vi "LSMcontroller_v61_updatedROIselection.vi"() -> ()   [LabVIEW 2015] (continued)
                    n4179 = local read "srateAODOtt"() -> (w920:dbl)
                    n4180 = local read "srateAODOtt"() -> (w927:dbl)
                    n4181 = local read "continuous"() -> (w932:bool)
                    n4182 = local read "Angle ref"() -> (w917:dbl)
                    n4183 = local read "wavdet"() -> (w934:bool)
                    n4184 = local read "Vx-ref"() -> (w929:dbl)
                    n4185 = local read "Vy-ref"() -> (w931:dbl)
                    n4186 = local read "avpp"() -> (w930:i32)
                    n4187 = call "tt_timeandsamples.vi"("bin"=w924, "refreshtime"=w918, "srateAODOtt"=w921, "tot#ofsamples"=w926) -> ("refreshrate"=w922:dbl, "refreshbuffer"=w923:i32, "timetracecycles"=w928:i32)  [unwired: 5 in]
                    n4188 = local read "bin"() -> (w925:dbl)
                    n4189 = call "2pparameters.vi"("command"="get") -> ("params out"=w937:T11)  [unwired: 1 in]
                    n4190 = Bundle By Name(cluster=w937, "Drawing Mode"=w910, "measpoints"=w926, "tt_cycles"=w928, "refreshbuffer"=w923, "refreshrate"=w922, "Vx-ref"=w929, "Vy-ref"=w931, "srate"=w920, "finite"=w933, "cont"=w932, "wavdet"=w934, "avpp"=w930, "srateAODO"=w927, "bufferAI"=w923, "bin"=w925, "Angle Img"=w917, "Vxminref"=w916, "Vxmaxref"=w915, "Vyminref"=w914, "Vymaxref"=w913, "Xpixels Img"=w912, "Ypixels Img"=w911, "Pel"=w909, "Vz-reset"=0.0, "AIoverride"=w907, "type"="Lifetime (contour)") -> (w935:T11)
                    n4191 = Reciprocal(x=w922) -> (1/x=w919:dbl)
                    n4192 = local write "refreshtime"(w919) -> ()
                    n4193 = call "2pparameters.vi"("Params in"=w935, "command"="set") -> ()  [unwired: 1 out]
                  }
                  frame "X-Y-Z-t movie" {
                  }
                  frame "linescan" {
                  }
                  frame "Timetrace" {
                    n4194 = local read "Vy-min draw"() -> (w947:dbl)
                    n4195 = local read "Vy-max draw"() -> (w946:dbl)
                    n4196 = local read "Vx-min draw"() -> (w949:dbl)
                    n4197 = local read "Vx-max draw"() -> (w948:dbl)
                    n4198 = local read "xpixels ref"() -> (w945:i32)
                    n4199 = local read "ypixels ref"() -> (w944:i32)
                    n4200 = local read "ROI Type"() -> (w943:u16)
                    n4201 = local read "srateAODOtt"() -> (w954:dbl)
                    n4202 = local read "# of frames"() -> (w959:i32)
                    n4203 = local read "refreshtime"() -> (w951:dbl)
                    n4204 = local read "Pel"() -> (w942:dbl)
                    n4205 = local read "bin"() -> (w957:dbl)
                    n4206 = local read "Override AI buffer"() -> (w940:bool)
                    n4207 = local read "finite samples"() -> (w966:bool)
                    n4208 = local read "srateAODOtt"() -> (w953:dbl)
                    n4209 = local read "srateAODOtt"() -> (w960:dbl)
                    n4210 = local read "continuous"() -> (w965:bool)
                    n4211 = local read "Angle ref"() -> (w950:dbl)
                    n4212 = local read "wavdet"() -> (w967:bool)
                    n4213 = local read "Vx-ref"() -> (w962:dbl)
                    n4214 = local read "Vy-ref"() -> (w964:dbl)
                    n4215 = local read "avpp"() -> (w963:i32)
                    n4216 = call "tt_timeandsamples.vi"("bin"=w957, "refreshtime"=w951, "srateAODOtt"=w954, "tot#ofsamples"=w959) -> ("refreshrate"=w955:dbl, "refreshbuffer"=w956:i32, "timetracecycles"=w961:i32)  [unwired: 5 in]
                    n4217 = local read "bin"() -> (w958:dbl)
                    n4218 = call "2pparameters.vi"("command"="get") -> ("params out"=w970:T11)  [unwired: 1 in]
                    n4219 = Bundle By Name(cluster=w970, "Drawing Mode"=w943, "measpoints"=w959, "tt_cycles"=w961, "refreshbuffer"=w956, "refreshrate"=w955, "Vx-ref"=w962, "Vy-ref"=w964, "srate"=w953, "finite"=w966, "cont"=w965, "wavdet"=w967, "avpp"=w963, "srateAODO"=w960, "bufferAI"=w956, "bin"=w958, "Angle Img"=w950, "Vxminref"=w949, "Vxmaxref"=w948, "Vyminref"=w947, "Vymaxref"=w946, "Xpixels Img"=w945, "Ypixels Img"=w944, "Pel"=w942, "Vz-reset"=0.0, "AIoverride"=w940, "type"="Timetrace") -> (w968:T11)
                    n4220 = Reciprocal(x=w955) -> (1/x=w952:dbl)
                    n4221 = local write "refreshtime"(w952) -> ()
                    n4222 = call "2pparameters.vi"("Params in"=w968, "command"="set") -> ()  [unwired: 1 out]
                  }
                  frame "Lifetime (point)" {
                  }
                }
              }
              frame #1 {
                w973 = FALSE ("wavdet")
                n4223 = call "2pparameters.vi"("command"="get") -> ("params out"=w977:T11)  [unwired: 1 in]
                n4224 = Bundle By Name(cluster=w977, "finite"=w973, "cont"=w973, "wavdet"=TRUE) -> (w974:T11)
                n4225 = call "2pparameters.vi"("Params in"=w974, "command"="set") -> ()  [unwired: 1 out]
              }
              frame #2 {
                n4226 = local read "DO channels"() -> (w982:u16)
                n4227 = call "2pparameters.vi"("command"="get") -> ("params out"=w984:T11)  [unwired: 1 in]
                n4228 = Unbundle By Name(w984) -> ("aDO"=w983:u32[])
                n4229 = Search 1D Array(1D array=w983, element=w982) -> (index of element=w980:i32)  [unwired: 1 in]
                n4230 = Greater?(x=w980, y=-1) -> (0:w979:bool)
                n4231 = case shown="True" w979 {
                  tunnel: w980 -> [_ w993]
                  frame False {
                  }
                  frame True {
                    n4232 = local read "Meastab"() -> (w987:enum32{"X-Y Image", "Linescan", "Timetrace"})
                    n4233 = local read "Digital padding value"() -> (w988:dbl)
                    n4234 = local read "Digital time offset (s)"() -> (w989:dbl)
                    n4235 = case shown="\"Timetrace\"" w987 {
                      tunnel: [w994 w995] -> w986
                      frame "X-Y Image", Default {
                        n4236 = local read "Sampling rate"() -> (w994:dbl)
                      }
                      frame "Timetrace" {
                        n4237 = local read "srateAODOtt"() -> (w995:dbl)
                      }
                    }
                    n4238 = local read "Digital Freq (Hz)"() -> (w991:dbl)
                    n4239 = local read "Digital phase (s)"() -> (w990:dbl)
                    n4240 = local read "Digital DC (%)"() -> (w992:dbl)
                    n4241 = call "replace DO wf param.vi"("Digital Freq (Hz)"=w991, "Digital DC (%)"=w992, "Digital phase"=w990, "Sampling frequency (Hz)"=w986, "Digital time offset (s)"=w989, "index of DO wave"=w993, "padding value"=w988) -> ()  [unwired: 4 in]
                  }
                }
              }
              frame #3 {
                n4242 = case shown="True" w996 {
                  tunnel: w997 -> [_ w1004]
                  frame False {
                  }
                  frame True {
                    n4243 = local read "Meastab"() -> (w1001:enum32{"X-Y Image", "Linescan", "Timetrace"})
                    n4244 = call "waveformparamsv2.vi"("command"="get") -> ("Params out"=w1020:T15)  [unwired: 4 in, 2 out]
                    n4245 = Unbundle By Name(w1020) -> ("DO parameters"=w1019:T18)
                    n4246 = property on="refwf" class="Ring (strict)"() -> ("RingText.Text"=w1026:string)  [unwired: 2 in, 2 out]
                    n4247 = case shown="\"Timetrace\"" w1001 {
                      tunnel: [w1027 w1028] -> w1000
                      frame "X-Y Image", Default {
                        n4248 = local read "Sampling rate"() -> (w1027:dbl)
                      }
                      frame "Timetrace" {
                        n4249 = local read "srateAODOtt"() -> (w1028:dbl)
                      }
                    }
                    n4250 = call "waveformsAObuffer.vi"("command"="get") -> ("AO wf out"=w1024:waveform(dbl)[])  [unwired: 1 in]
                    n4251 = call "waveformsDObuffer.vi"("command"="get") -> ("DO wf out"=w1022:digitalwaveform[])  [unwired: 1 in]
                    n4252 = call "referfencesize.vi"("Digital waveforms in"=w1022, "Analog waveforms in"=w1024, "reference waveforms to"=w1026) -> ("number of samples"=w1017:i32)  [unwired: 2 in]
                    n4253 = Index Array(array=w1019, index=w1004) -> (element=w1018:T19)
                    n4254 = call "waveformsDObuffer.vi"("command"="get") -> ("DO wf out"=w1014:digitalwaveform[])  [unwired: 1 in]
                    n4255 = call "simple digital from wf params.vi"("waveform params"=w1018, "number of samples"=w1017) -> ("digital waveform"=w1016:digitalwaveform)
                    n4256 = property on="refwf" class="Ring (strict)"() -> ("RingText.Text"=w1006:string)  [unwired: 2 in, 2 out]
                    n4257 = Replace Array Subset(array=w1014, new element=w1016, index=w1004) -> (w1005:digitalwaveform[])
                    n4258 = call "waveformsAObuffer.vi"("command"="get") -> ("AO wf out"=w1013:waveform(dbl)[])  [unwired: 1 in]
                    n4259 = local read "wavdet"() -> (w1003:bool)
                    n4260 = call "correctwaveformsizetemp.vi"("new sampling frequency (Hz)"=w1000, "start"=FALSE, "reference waveforms to"=w1006, "Analog waveforms in"=w1013, "stop"=FALSE, "Digital waveforms in"=w1005) -> ("analog wf out"=w1009:waveform(dbl)[], "Digital wf out"=w1007:digitalwaveform[], "measpoints"=w1002:i32)
                    n4261 = local write "Analog Lines Plot"(w1009) -> ()
                    n4262 = call "GetNumCamFramesv2.vi"("Digital Waveform Graph"=w1007) -> ("Numeric"=w1008:i32)  [unwired: 10 in]
                    n4263 = local write "Digital Lines Plot"(w1007) -> ()
                    n4264 = case shown="True" w1003 {
                      tunnel: w1002 -> [_ w1029]
                      frame False {
                      }
                      frame True {
                        n4265 = local write "# of frames"(w1029) -> ()
                      }
                    }
                    n4266 = call "waveformsAObuffer.vi"("AO wf in"=w1009, "command"="set") -> ()  [unwired: 1 out]
                    n4267 = call "waveformsDObuffer.vi"("DO wf in"=w1007, "command"="set") -> ()  [unwired: 1 out]
                    n4268 = local write "Total Camera Frames"(w1008) -> ()
                  }
                }
              }
              frame #4 {
                n4269 = local read "finite samples"() -> (w1030:bool)
                n4270 = local read "continuous"() -> (w1031:bool)
                n4271 = local read "wavdet"() -> (w1032:bool)
                n4272 = call "2pparameters.vi"("command"="get") -> ("params out"=w1035:T11)  [unwired: 1 in]
                n4273 = Bundle By Name(cluster=w1035, "finite"=w1030, "cont"=w1031, "wavdet"=w1032) -> (w1033:T11)
                n4274 = call "2pparameters.vi"("Params in"=w1033, "command"="set") -> ()  [unwired: 1 out]
              }
            }
          }
          event "refwf": Value Change {
            n4275 = event-data() -> ()  [unwired: 1 in, 6 out]
            n4276 = stacked-sequence {
              frame #0 {
                n4277 = local read "Measurement"() -> (w1037:T4)
                n4278 = case shown="\"X-Y-t movie\", Default" w1037 {
                  frame "X-Y-t movie", Default {
                    n4279 = local read "avpp"() -> (w1058:i32)
                    n4280 = local read "Angle ref"() -> (w1057:dbl)
                    n4281 = local read "ROI Type"() -> (w1056:u16)
                    n4282 = local read "xpixels ref"() -> (w1053:i32)
                    n4283 = local read "Vx-min ref"() -> (w1052:dbl)
                    n4284 = local read "Vx-max ref"() -> (w1051:dbl)
                    n4285 = local read "ypixels ref"() -> (w1049:i32)
                    n4286 = local read "Vy-min ref"() -> (w1050:dbl)
                    n4287 = local read "Vy-max ref"() -> (w1046:dbl)
                    n4288 = local read "Sampling rate"() -> (w1040:dbl)
                    n4289 = local read "finite samples"() -> (w1041:bool)
                    n4290 = local read "continuous"() -> (w1044:bool)
                    n4291 = local read "wavdet"() -> (w1045:bool)
                    n4292 = local read "# of frames"() -> (w1043:i32)
                    n4293 = local read "maxbufferAI"() -> (w1042:i32)
                    n4294 = local read "Override AI buffer"() -> (w1038:bool)
                    n4295 = call "2pparameters.vi"("command"="get") -> ("params out"=w1055:T11)  [unwired: 1 in]
                    n4296 = Bundle By Name(cluster=w1055, "type"="X-Y-t movie", "avpp"=w1058, "Angle Img"=w1057, "Xpixels Img"=w1053, "Vx-min Img"=w1052, "VX-max Img"=w1051, "Ypixels Img"=w1049, "Vy-min Img"=w1050, "Vy-max Img"=w1046, "srate"=w1040, "srate Img"=w1040, "finite"=w1041, "cont"=w1044, "wavdet"=w1045, "measpoints"=w1043, "maxbufferAI"=w1042, "Drawing Mode"=w1056, "Vz-reset"=0.0, "AIoverride"=w1038) -> (w1047:T11)
                    n4297 = call "2pparameters.vi"("Params in"=w1047, "command"="set") -> ()  [unwired: 1 out]
                  }
                  frame "X-Y-Z stack" {
                    n4298 = call "2pparameters.vi"("command"="get") -> ("params out"=w1062:T11)  [unwired: 1 in]
                    n4299 = Bundle By Name(cluster=w1062, "type"="X-Y-Z stack") -> (w1060:T11)
                    n4300 = call "2pparameters.vi"("Params in"=w1060, "command"="set") -> ()  [unwired: 1 out]
                  }
                  frame "Lifetime (scan)" {
                    n4301 = call "2pparameters.vi"("command"="get") -> ("params out"=w1067:T11)  [unwired: 1 in]
                    n4302 = Bundle By Name(cluster=w1067, "type"="Lifetime (scan)") -> (w1065:T11)
                    n4303 = call "2pparameters.vi"("Params in"=w1065, "command"="set") -> ()  [unwired: 1 out]
                  }
                  frame "Lifetime (contour)" {
                    n4304 = local read "Vy-min draw"() -> (w1077:dbl)
                    n4305 = local read "Vy-max draw"() -> (w1076:dbl)
                    n4306 = local read "Vx-min draw"() -> (w1079:dbl)
                    n4307 = local read "Vx-max draw"() -> (w1078:dbl)
                    n4308 = local read "xpixels ref"() -> (w1075:i32)
                    n4309 = local read "ypixels ref"() -> (w1074:i32)
                    n4310 = local read "ROI Type"() -> (w1073:u16)
                    n4311 = local read "srateAODOtt"() -> (w1084:dbl)
                    n4312 = local read "# of frames"() -> (w1089:i32)
                    n4313 = local read "refreshtime"() -> (w1081:dbl)
                    n4314 = local read "Pel"() -> (w1072:dbl)
                    n4315 = local read "bin"() -> (w1087:dbl)
                    n4316 = local read "Override AI buffer"() -> (w1070:bool)
                    n4317 = local read "finite samples"() -> (w1096:bool)
                    n4318 = local read "srateAODOtt"() -> (w1083:dbl)
                    n4319 = local read "srateAODOtt"() -> (w1090:dbl)
                    n4320 = local read "continuous"() -> (w1095:bool)
                    n4321 = local read "Angle ref"() -> (w1080:dbl)
                    n4322 = local read "wavdet"() -> (w1097:bool)
                    n4323 = local read "Vx-ref"() -> (w1092:dbl)
                    n4324 = local read "Vy-ref"() -> (w1094:dbl)
                    n4325 = local read "avpp"() -> (w1093:i32)
                    n4326 = call "tt_timeandsamples.vi"("bin"=w1087, "refreshtime"=w1081, "srateAODOtt"=w1084, "tot#ofsamples"=w1089) -> ("refreshrate"=w1085:dbl, "refreshbuffer"=w1086:i32, "timetracecycles"=w1091:i32)  [unwired: 5 in]
                    n4327 = local read "bin"() -> (w1088:dbl)
                    n4328 = call "2pparameters.vi"("command"="get") -> ("params out"=w1100:T11)  [unwired: 1 in]
                    n4329 = Bundle By Name(cluster=w1100, "Drawing Mode"=w1073, "measpoints"=w1089, "tt_cycles"=w1091, "refreshbuffer"=w1086, "refreshrate"=w1085, "Vx-ref"=w1092, "Vy-ref"=w1094, "srate"=w1083, "finite"=w1096, "cont"=w1095, "wavdet"=w1097, "avpp"=w1093, "srateAODO"=w1090, "bufferAI"=w1086, "bin"=w1088, "Angle Img"=w1080, "Vxminref"=w1079, "Vxmaxref"=w1078, "Vyminref"=w1077, "Vymaxref"=w1076, "Xpixels Img"=w1075, "Ypixels Img"=w1074, "Pel"=w1072, "Vz-reset"=0.0, "AIoverride"=w1070, "type"="Lifetime (contour)") -> (w1098:T11)
                    n4330 = Reciprocal(x=w1085) -> (1/x=w1082:dbl)
                    n4331 = local write "refreshtime"(w1082) -> ()
                    n4332 = call "2pparameters.vi"("Params in"=w1098, "command"="set") -> ()  [unwired: 1 out]
                  }
                  frame "X-Y-Z-t movie" {
                  }
                  frame "linescan" {
                  }
                  frame "Timetrace" {
                    n4333 = local read "Vy-min draw"() -> (w1110:dbl)
                    n4334 = local read "Vy-max draw"() -> (w1109:dbl)
                    n4335 = local read "Vx-min draw"() -> (w1112:dbl)
                    n4336 = local read "Vx-max draw"() -> (w1111:dbl)
                    n4337 = local read "xpixels ref"() -> (w1108:i32)
                    n4338 = local read "ypixels ref"() -> (w1107:i32)
                    n4339 = local read "ROI Type"() -> (w1106:u16)
                    n4340 = local read "srateAODOtt"() -> (w1117:dbl)
                    n4341 = local read "# of frames"() -> (w1122:i32)
                    n4342 = local read "refreshtime"() -> (w1114:dbl)
                    n4343 = local read "Pel"() -> (w1105:dbl)
                    n4344 = local read "bin"() -> (w1120:dbl)
                    n4345 = local read "Override AI buffer"() -> (w1103:bool)
                    n4346 = local read "finite samples"() -> (w1129:bool)
                    n4347 = local read "srateAODOtt"() -> (w1116:dbl)
                    n4348 = local read "srateAODOtt"() -> (w1123:dbl)
                    n4349 = local read "continuous"() -> (w1128:bool)
                    n4350 = local read "Angle ref"() -> (w1113:dbl)
                    n4351 = local read "wavdet"() -> (w1130:bool)
                    n4352 = local read "Vx-ref"() -> (w1125:dbl)
                    n4353 = local read "Vy-ref"() -> (w1127:dbl)
                    n4354 = local read "avpp"() -> (w1126:i32)
                    n4355 = call "tt_timeandsamples.vi"("bin"=w1120, "refreshtime"=w1114, "srateAODOtt"=w1117, "tot#ofsamples"=w1122) -> ("refreshrate"=w1118:dbl, "refreshbuffer"=w1119:i32, "timetracecycles"=w1124:i32)  [unwired: 5 in]
                    n4356 = local read "bin"() -> (w1121:dbl)
                    n4357 = call "2pparameters.vi"("command"="get") -> ("params out"=w1133:T11)  [unwired: 1 in]
                    n4358 = Bundle By Name(cluster=w1133, "Drawing Mode"=w1106, "measpoints"=w1122, "tt_cycles"=w1124, "refreshbuffer"=w1119, "refreshrate"=w1118, "Vx-ref"=w1125, "Vy-ref"=w1127, "srate"=w1116, "finite"=w1129, "cont"=w1128, "wavdet"=w1130, "avpp"=w1126, "srateAODO"=w1123, "bufferAI"=w1119, "bin"=w1121, "Angle Img"=w1113, "Vxminref"=w1112, "Vxmaxref"=w1111, "Vyminref"=w1110, "Vymaxref"=w1109, "Xpixels Img"=w1108, "Ypixels Img"=w1107, "Pel"=w1105, "Vz-reset"=0.0, "AIoverride"=w1103, "type"="Timetrace") -> (w1131:T11)
                    n4359 = Reciprocal(x=w1118) -> (1/x=w1115:dbl)
                    n4360 = local write "refreshtime"(w1115) -> ()
                    n4361 = call "2pparameters.vi"("Params in"=w1131, "command"="set") -> ()  [unwired: 1 out]
                  }
                  frame "Lifetime (point)" {
                  }
                }
              }
              frame #1 {
                w1136 = FALSE ("wavdet")
                n4362 = call "2pparameters.vi"("command"="get") -> ("params out"=w1140:T11)  [unwired: 1 in]
                n4363 = Bundle By Name(cluster=w1140, "finite"=w1136, "cont"=w1136, "wavdet"=TRUE) -> (w1137:T11)
                n4364 = call "2pparameters.vi"("Params in"=w1137, "command"="set") -> ()  [unwired: 1 out]
              }
              frame #2 {
                n4365 = local read "Meastab"() -> (w1145:enum32{"X-Y Image", "Linescan", "Timetrace"})
                n4366 = property on="refwf" class="Ring (strict)"() -> ("RingText.Text"=w1148:string)  [unwired: 2 in, 2 out]
                n4367 = case shown="\"Timetrace\"" w1145 {
                  tunnel: [w1158 w1159] -> w1144
                  frame "X-Y Image", Default {
                    n4368 = local read "Sampling rate"() -> (w1158:dbl)
                  }
                  frame "Timetrace" {
                    n4369 = local read "srateAODOtt"() -> (w1159:dbl)
                  }
                }
                n4370 = call "waveformsAObuffer.vi"("command"="get") -> ("AO wf out"=w1157:waveform(dbl)[])  [unwired: 1 in]
                n4371 = local read "wavdet"() -> (w1147:bool)
                n4372 = call "waveformsDObuffer.vi"("command"="get") -> ("DO wf out"=w1153:digitalwaveform[])  [unwired: 1 in]
                n4373 = call "correctwaveformsizetemp.vi"("new sampling frequency (Hz)"=w1144, "start"=FALSE, "reference waveforms to"=w1148, "Analog waveforms in"=w1157, "stop"=FALSE, "Digital waveforms in"=w1153) -> ("analog wf out"=w1151:waveform(dbl)[], "Digital wf out"=w1149:digitalwaveform[], "measpoints"=w1146:i32)
                n4374 = local write "Analog Lines Plot"(w1151) -> ()
                n4375 = call "GetNumCamFramesv2.vi"("Digital Waveform Graph"=w1149) -> ("Numeric"=w1150:i32)  [unwired: 10 in]
                n4376 = local write "Digital Lines Plot"(w1149) -> ()
                n4377 = call "waveformsDObuffer.vi"("DO wf in"=w1149, "command"="set") -> ()  [unwired: 1 out]
                n4378 = call "waveformsAObuffer.vi"("AO wf in"=w1151, "command"="set") -> ()  [unwired: 1 out]
                n4379 = local write "Total Camera Frames"(w1150) -> ()
                n4380 = case shown="True" w1147 {
                  tunnel: w1146 -> [_ w1160]
                  frame False {
                  }
                  frame True {
                    n4381 = local write "# of frames"(w1160) -> ()
                  }
                }
              }
              frame #3 {
                n4382 = local read "finite samples"() -> (w1161:bool)
                n4383 = local read "continuous"() -> (w1162:bool)
                n4384 = local read "wavdet"() -> (w1163:bool)
                n4385 = call "2pparameters.vi"("command"="get") -> ("params out"=w1166:T11)  [unwired: 1 in]
                n4386 = Bundle By Name(cluster=w1166, "finite"=w1161, "cont"=w1162, "wavdet"=w1163) -> (w1164:T11)
                n4387 = call "2pparameters.vi"("Params in"=w1164, "command"="set") -> ()  [unwired: 1 out]
              }
            }
          }
          event "Start amplitude (V)", "Cycles", "Baseline (V)", "Step size (V)", "DC (%)", "Period (ms)", "Repeats", "Pulses", "phase shift (ms)": Value Change {
            n4388 = event-data() -> ()  [unwired: 1 in, 6 out]
            n4389 = stacked-sequence {
              seq-local: [_ _ w1274 _ _] -> [_ _ _ w1296 _]
              seq-local: [_ _ w1273 _ _] -> [_ _ _ w1295 _]
              frame #0 {
                n4390 = local read "Measurement"() -> (w1168:T4)
                n4391 = case shown="\"X-Y-t movie\", Default" w1168 {
                  frame "X-Y-t movie", Default {
                    n4392 = local read "avpp"() -> (w1189:i32)
                    n4393 = local read "Angle ref"() -> (w1188:dbl)
                    n4394 = local read "ROI Type"() -> (w1187:u16)
                    n4395 = local read "xpixels ref"() -> (w1184:i32)
                    n4396 = local read "Vx-min ref"() -> (w1183:dbl)
                    n4397 = local read "Vx-max ref"() -> (w1182:dbl)
                    n4398 = local read "ypixels ref"() -> (w1180:i32)
                    n4399 = local read "Vy-min ref"() -> (w1181:dbl)
                    n4400 = local read "Vy-max ref"() -> (w1177:dbl)
                    n4401 = local read "Sampling rate"() -> (w1171:dbl)
                    n4402 = local read "finite samples"() -> (w1172:bool)
                    n4403 = local read "continuous"() -> (w1175:bool)
                    n4404 = local read "wavdet"() -> (w1176:bool)
                    n4405 = local read "# of frames"() -> (w1174:i32)
                    n4406 = local read "maxbufferAI"() -> (w1173:i32)
                    n4407 = local read "Override AI buffer"() -> (w1169:bool)
                    n4408 = call "2pparameters.vi"("command"="get") -> ("params out"=w1186:T11)  [unwired: 1 in]
                    n4409 = Bundle By Name(cluster=w1186, "type"="X-Y-t movie", "avpp"=w1189, "Angle Img"=w1188, "Xpixels Img"=w1184, "Vx-min Img"=w1183, "VX-max Img"=w1182, "Ypixels Img"=w1180, "Vy-min Img"=w1181, "Vy-max Img"=w1177, "srate"=w1171, "srate Img"=w1171, "finite"=w1172, "cont"=w1175, "wavdet"=w1176, "measpoints"=w1174, "maxbufferAI"=w1173, "Drawing Mode"=w1187, "Vz-reset"=0.0, "AIoverride"=w1169) -> (w1178:T11)
                    n4410 = call "2pparameters.vi"("Params in"=w1178, "command"="set") -> ()  [unwired: 1 out]
                  }
                  frame "X-Y-Z stack" {
                    n4411 = call "2pparameters.vi"("command"="get") -> ("params out"=w1193:T11)  [unwired: 1 in]
                    n4412 = Bundle By Name(cluster=w1193, "type"="X-Y-Z stack") -> (w1191:T11)
                    n4413 = call "2pparameters.vi"("Params in"=w1191, "command"="set") -> ()  [unwired: 1 out]
                  }
                  frame "Lifetime (scan)" {
                    n4414 = call "2pparameters.vi"("command"="get") -> ("params out"=w1198:T11)  [unwired: 1 in]
                    n4415 = Bundle By Name(cluster=w1198, "type"="Lifetime (scan)") -> (w1196:T11)
                    n4416 = call "2pparameters.vi"("Params in"=w1196, "command"="set") -> ()  [unwired: 1 out]
                  }
                  frame "Lifetime (contour)" {
                    n4417 = local read "Vy-min draw"() -> (w1208:dbl)
                    n4418 = local read "Vy-max draw"() -> (w1207:dbl)
                    n4419 = local read "Vx-min draw"() -> (w1210:dbl)
                    n4420 = local read "Vx-max draw"() -> (w1209:dbl)
                    n4421 = local read "xpixels ref"() -> (w1206:i32)
                    n4422 = local read "ypixels ref"() -> (w1205:i32)
                    n4423 = local read "ROI Type"() -> (w1204:u16)
                    n4424 = local read "srateAODOtt"() -> (w1215:dbl)
                    n4425 = local read "# of frames"() -> (w1220:i32)
                    n4426 = local read "refreshtime"() -> (w1212:dbl)
                    n4427 = local read "Pel"() -> (w1203:dbl)
                    n4428 = local read "bin"() -> (w1218:dbl)
                    n4429 = local read "Override AI buffer"() -> (w1201:bool)
                    n4430 = local read "finite samples"() -> (w1227:bool)
                    n4431 = local read "srateAODOtt"() -> (w1214:dbl)
                    n4432 = local read "srateAODOtt"() -> (w1221:dbl)
                    n4433 = local read "continuous"() -> (w1226:bool)
                    n4434 = local read "Angle ref"() -> (w1211:dbl)
                    n4435 = local read "wavdet"() -> (w1228:bool)
                    n4436 = local read "Vx-ref"() -> (w1223:dbl)
                    n4437 = local read "Vy-ref"() -> (w1225:dbl)
                    n4438 = local read "avpp"() -> (w1224:i32)
                    n4439 = call "tt_timeandsamples.vi"("bin"=w1218, "refreshtime"=w1212, "srateAODOtt"=w1215, "tot#ofsamples"=w1220) -> ("refreshrate"=w1216:dbl, "refreshbuffer"=w1217:i32, "timetracecycles"=w1222:i32)  [unwired: 5 in]
                    n4440 = local read "bin"() -> (w1219:dbl)
                    n4441 = call "2pparameters.vi"("command"="get") -> ("params out"=w1231:T11)  [unwired: 1 in]
                    n4442 = Bundle By Name(cluster=w1231, "Drawing Mode"=w1204, "measpoints"=w1220, "tt_cycles"=w1222, "refreshbuffer"=w1217, "refreshrate"=w1216, "Vx-ref"=w1223, "Vy-ref"=w1225, "srate"=w1214, "finite"=w1227, "cont"=w1226, "wavdet"=w1228, "avpp"=w1224, "srateAODO"=w1221, "bufferAI"=w1217, "bin"=w1219, "Angle Img"=w1211, "Vxminref"=w1210, "Vxmaxref"=w1209, "Vyminref"=w1208, "Vymaxref"=w1207, "Xpixels Img"=w1206, "Ypixels Img"=w1205, "Pel"=w1203, "Vz-reset"=0.0, "AIoverride"=w1201, "type"="Lifetime (contour)") -> (w1229:T11)
                    n4443 = Reciprocal(x=w1216) -> (1/x=w1213:dbl)
                    n4444 = local write "refreshtime"(w1213) -> ()
                    n4445 = call "2pparameters.vi"("Params in"=w1229, "command"="set") -> ()  [unwired: 1 out]
                  }
                  frame "X-Y-Z-t movie" {
                  }
                  frame "linescan" {
                  }
                  frame "Timetrace" {
                    n4446 = local read "Vy-min draw"() -> (w1241:dbl)
                    n4447 = local read "Vy-max draw"() -> (w1240:dbl)
                    n4448 = local read "Vx-min draw"() -> (w1243:dbl)
                    n4449 = local read "Vx-max draw"() -> (w1242:dbl)
                    n4450 = local read "xpixels ref"() -> (w1239:i32)
                    n4451 = local read "ypixels ref"() -> (w1238:i32)
                    n4452 = local read "ROI Type"() -> (w1237:u16)
                    n4453 = local read "srateAODOtt"() -> (w1248:dbl)
                    n4454 = local read "# of frames"() -> (w1253:i32)
                    n4455 = local read "refreshtime"() -> (w1245:dbl)
                    n4456 = local read "Pel"() -> (w1236:dbl)
                    n4457 = local read "bin"() -> (w1251:dbl)
                    n4458 = local read "Override AI buffer"() -> (w1234:bool)
                    n4459 = local read "finite samples"() -> (w1260:bool)
                    n4460 = local read "srateAODOtt"() -> (w1247:dbl)
                    n4461 = local read "srateAODOtt"() -> (w1254:dbl)
                    n4462 = local read "continuous"() -> (w1259:bool)
                    n4463 = local read "Angle ref"() -> (w1244:dbl)
                    n4464 = local read "wavdet"() -> (w1261:bool)
                    n4465 = local read "Vx-ref"() -> (w1256:dbl)
                    n4466 = local read "Vy-ref"() -> (w1258:dbl)
                    n4467 = local read "avpp"() -> (w1257:i32)
                    n4468 = call "tt_timeandsamples.vi"("bin"=w1251, "refreshtime"=w1245, "srateAODOtt"=w1248, "tot#ofsamples"=w1253) -> ("refreshrate"=w1249:dbl, "refreshbuffer"=w1250:i32, "timetracecycles"=w1255:i32)  [unwired: 5 in]
                    n4469 = local read "bin"() -> (w1252:dbl)
                    n4470 = call "2pparameters.vi"("command"="get") -> ("params out"=w1264:T11)  [unwired: 1 in]
                    n4471 = Bundle By Name(cluster=w1264, "Drawing Mode"=w1237, "measpoints"=w1253, "tt_cycles"=w1255, "refreshbuffer"=w1250, "refreshrate"=w1249, "Vx-ref"=w1256, "Vy-ref"=w1258, "srate"=w1247, "finite"=w1260, "cont"=w1259, "wavdet"=w1261, "avpp"=w1257, "srateAODO"=w1254, "bufferAI"=w1250, "bin"=w1252, "Angle Img"=w1244, "Vxminref"=w1243, "Vxmaxref"=w1242, "Vyminref"=w1241, "Vymaxref"=w1240, "Xpixels Img"=w1239, "Ypixels Img"=w1238, "Pel"=w1236, "Vz-reset"=0.0, "AIoverride"=w1234, "type"="Timetrace") -> (w1262:T11)
                    n4472 = Reciprocal(x=w1249) -> (1/x=w1246:dbl)
                    n4473 = local write "refreshtime"(w1246) -> ()
                    n4474 = call "2pparameters.vi"("Params in"=w1262, "command"="set") -> ()  [unwired: 1 out]
                  }
                  frame "Lifetime (point)" {
                  }
                }
              }
              frame #1 {
                w1267 = FALSE ("wavdet")
                n4475 = call "2pparameters.vi"("command"="get") -> ("params out"=w1271:T11)  [unwired: 1 in]
                n4476 = Bundle By Name(cluster=w1271, "finite"=w1267, "cont"=w1267, "wavdet"=TRUE) -> (w1268:T11)
                n4477 = call "2pparameters.vi"("Params in"=w1268, "command"="set") -> ()  [unwired: 1 out]
              }
              frame #2 {
                n4478 = local read "AO channels"() -> (w1276:u32)
                n4479 = call "2pparameters.vi"("command"="get") -> ("params out"=w1278:T11)  [unwired: 1 in]
                n4480 = Unbundle By Name(w1278) -> ("aAO"=w1277:u32[])
                n4481 = Search 1D Array(1D array=w1277, element=w1276) -> (index of element=w1274:i32)  [unwired: 1 in]
                n4482 = Greater?(x=w1274, y=-1) -> (0:w1273:bool)
                n4483 = case shown="True" w1273 {
                  tunnel: w1274 -> [_ w1292]
                  frame False {
                  }
                  frame True {
                    n4484 = local read "Meastab"() -> (w1281:enum32{"X-Y Image", "Linescan", "Timetrace"})
                    n4485 = case shown="\"Timetrace\"" w1281 {
                      tunnel: [w1293 w1294] -> w1280
                      frame "X-Y Image", Default {
                        n4486 = local read "Sampling rate"() -> (w1293:dbl)
                      }
                      frame "Timetrace" {
                        n4487 = local read "srateAODOtt"() -> (w1294:dbl)
                      }
                    }
                    n4488 = local read "Start amplitude (V)"() -> (w1289:dbl)
                    n4489 = local read "phase shift (ms)"() -> (w1284:dbl)
                    n4490 = local read "Step size (V)"() -> (w1287:dbl)
                    n4491 = local read "Baseline (V)"() -> (w1288:dbl)
                    n4492 = local read "Period (ms)"() -> (w1285:dbl)
                    n4493 = local read "padding value"() -> (w1282:dbl)
                    n4494 = local read "Repeats"() -> (w1291:dbl)
                    n4495 = local read "Cycles"() -> (w1290:dbl)
                    n4496 = local read "DC (%)"() -> (w1286:dbl)
                    n4497 = local read "Pulses"() -> (w1283:dbl)
                    n4498 = call "replace AO square wf param.vi"("Baseline (V)"=w1288, "Start amplitude (V)"=w1289, "Cycles"=w1290, "Repeats"=w1291, "index of AO wave"=w1292, "Step size (V)"=w1287, "DC (%)"=w1286, "Sampling frequency (Hz)"=w1280, "Period (ms)"=w1285, "Cycle length (s)"=w1284, "Pulses"=w1283, "padding value"=w1282) -> ()  [unwired: 4 in]
                  }
                }
              }
              frame #3 {
                n4499 = case shown="True" w1295 {
                  tunnel: w1296 -> [_ w1304]
                  frame False {
                  }
                  frame True {
                    n4500 = call "waveformparamsv2.vi"("command"="get") -> ("Params out"=w1318:T15)  [unwired: 4 in, 2 out]
                    n4501 = Unbundle By Name(w1318) -> ("AO parameters"=w1317:T16)
                    n4502 = local read "Meastab"() -> (w1299:enum32{"X-Y Image", "Linescan", "Timetrace"})
                    n4503 = case shown="\"Timetrace\"" w1299 {
                      tunnel: [w1320 w1321] -> w1308
                      frame "X-Y Image", Default {
                        n4504 = local read "Sampling rate"() -> (w1320:dbl)
                      }
                      frame "Timetrace" {
                        n4505 = local read "srateAODOtt"() -> (w1321:dbl)
                      }
                    }
                    n4506 = Index Array(array=w1317, index=w1304) -> (element=w1306:T17)
                    n4507 = call "waveformsAObuffer.vi"("command"="get") -> ("AO wf out"=w1305:waveform(dbl)[])  [unwired: 1 in]
                    n4508 = call "generateRampedSquareWave_fromAOparameters.vi"("AO params"=w1306) -> ("Waveform"=w1303:waveform(dbl))  [unwired: 1 out]
                    n4509 = property on="refwf" class="Ring (strict)"() -> ("RingText.Text"=w1307:string)  [unwired: 2 in, 2 out]
                    n4510 = Replace Array Subset(array=w1305, new element=w1303, index=w1304) -> (w1302:waveform(dbl)[])
                    n4511 = call "waveformsDObuffer.vi"("command"="get") -> ("DO wf out"=w1313:digitalwaveform[])  [unwired: 1 in]
                    n4512 = call "correctwaveformsizetemp.vi"("new sampling frequency (Hz)"=w1308, "start"=FALSE, "reference waveforms to"=w1307, "Analog waveforms in"=w1302, "stop"=FALSE, "Digital waveforms in"=w1313) -> ("analog wf out"=w1311:waveform(dbl)[], "Digital wf out"=w1309:digitalwaveform[], "measpoints"=w1300:i32)
                    n4513 = local read "wavdet"() -> (w1301:bool)
                    n4514 = local write "Analog Lines Plot"(w1311) -> ()
                    n4515 = call "GetNumCamFramesv2.vi"("Digital Waveform Graph"=w1309) -> ("Numeric"=w1310:i32)  [unwired: 10 in]
                    n4516 = local write "Digital Lines Plot"(w1309) -> ()
                    n4517 = call "waveformsAObuffer.vi"("AO wf in"=w1311, "command"="set") -> ()  [unwired: 1 out]
                    n4518 = call "waveformsDObuffer.vi"("DO wf in"=w1309, "command"="set") -> ()  [unwired: 1 out]
                    n4519 = local write "Total Camera Frames"(w1310) -> ()
                    n4520 = case shown="True" w1301 {
                      tunnel: w1300 -> [_ w1322]
                      frame False {
                      }
                      frame True {
                        n4521 = local write "# of frames"(w1322) -> ()
                      }
                    }
                  }
                }
              }
              frame #4 {
                n4522 = local read "finite samples"() -> (w1323:bool)
                n4523 = local read "continuous"() -> (w1324:bool)
                n4524 = local read "wavdet"() -> (w1325:bool)
                n4525 = call "2pparameters.vi"("command"="get") -> ("params out"=w1328:T11)  [unwired: 1 in]
                n4526 = Bundle By Name(cluster=w1328, "finite"=w1323, "cont"=w1324, "wavdet"=w1325) -> (w1326:T11)
                n4527 = call "2pparameters.vi"("Params in"=w1326, "command"="set") -> ()  [unwired: 1 out]
              }
            }
          }
          event "Amplitude (V)", "Offset (V)", "Frequency", "Tri Repeats": Value Change {
            n4528 = event-data() -> ()  [unwired: 1 in, 6 out]
            n4529 = stacked-sequence {
              seq-local: [_ _ w1436 _ _] -> [_ _ _ w1454 _]
              seq-local: [_ _ w1435 _ _] -> [_ _ _ w1453 _]
              frame #0 {
                n4530 = local read "Measurement"() -> (w1330:T4)
                n4531 = case shown="\"X-Y-t movie\", Default" w1330 {
                  frame "X-Y-t movie", Default {
                    n4532 = local read "avpp"() -> (w1351:i32)
                    n4533 = local read "Angle ref"() -> (w1350:dbl)
                    n4534 = local read "ROI Type"() -> (w1349:u16)
                    n4535 = local read "xpixels ref"() -> (w1346:i32)
                    n4536 = local read "Vx-min ref"() -> (w1345:dbl)
                    n4537 = local read "Vx-max ref"() -> (w1344:dbl)
                    n4538 = local read "ypixels ref"() -> (w1342:i32)
                    n4539 = local read "Vy-min ref"() -> (w1343:dbl)
                    n4540 = local read "Vy-max ref"() -> (w1339:dbl)
                    n4541 = local read "Sampling rate"() -> (w1333:dbl)
                    n4542 = local read "finite samples"() -> (w1334:bool)
                    n4543 = local read "continuous"() -> (w1337:bool)
                    n4544 = local read "wavdet"() -> (w1338:bool)
                    n4545 = local read "# of frames"() -> (w1336:i32)
                    n4546 = local read "maxbufferAI"() -> (w1335:i32)
                    n4547 = local read "Override AI buffer"() -> (w1331:bool)
                    n4548 = call "2pparameters.vi"("command"="get") -> ("params out"=w1348:T11)  [unwired: 1 in]
                    n4549 = Bundle By Name(cluster=w1348, "type"="X-Y-t movie", "avpp"=w1351, "Angle Img"=w1350, "Xpixels Img"=w1346, "Vx-min Img"=w1345, "VX-max Img"=w1344, "Ypixels Img"=w1342, "Vy-min Img"=w1343, "Vy-max Img"=w1339, "srate"=w1333, "srate Img"=w1333, "finite"=w1334, "cont"=w1337, "wavdet"=w1338, "measpoints"=w1336, "maxbufferAI"=w1335, "Drawing Mode"=w1349, "Vz-reset"=0.0, "AIoverride"=w1331) -> (w1340:T11)
                    n4550 = call "2pparameters.vi"("Params in"=w1340, "command"="set") -> ()  [unwired: 1 out]
                  }
                  frame "X-Y-Z stack" {
                    n4551 = call "2pparameters.vi"("command"="get") -> ("params out"=w1355:T11)  [unwired: 1 in]
                    n4552 = Bundle By Name(cluster=w1355, "type"="X-Y-Z stack") -> (w1353:T11)
                    n4553 = call "2pparameters.vi"("Params in"=w1353, "command"="set") -> ()  [unwired: 1 out]
                  }
                  frame "Lifetime (scan)" {
                    n4554 = call "2pparameters.vi"("command"="get") -> ("params out"=w1360:T11)  [unwired: 1 in]
                    n4555 = Bundle By Name(cluster=w1360, "type"="Lifetime (scan)") -> (w1358:T11)
                    n4556 = call "2pparameters.vi"("Params in"=w1358, "command"="set") -> ()  [unwired: 1 out]
                  }
                  frame "Lifetime (contour)" {
                    n4557 = local read "Vy-min draw"() -> (w1370:dbl)
                    n4558 = local read "Vy-max draw"() -> (w1369:dbl)
                    n4559 = local read "Vx-min draw"() -> (w1372:dbl)
                    n4560 = local read "Vx-max draw"() -> (w1371:dbl)
                    n4561 = local read "xpixels ref"() -> (w1368:i32)
                    n4562 = local read "ypixels ref"() -> (w1367:i32)
                    n4563 = local read "ROI Type"() -> (w1366:u16)
                    n4564 = local read "srateAODOtt"() -> (w1377:dbl)
                    n4565 = local read "# of frames"() -> (w1382:i32)
                    n4566 = local read "refreshtime"() -> (w1374:dbl)
                    n4567 = local read "Pel"() -> (w1365:dbl)
                    n4568 = local read "bin"() -> (w1380:dbl)
                    n4569 = local read "Override AI buffer"() -> (w1363:bool)
                    n4570 = local read "finite samples"() -> (w1389:bool)
                    n4571 = local read "srateAODOtt"() -> (w1376:dbl)
                    n4572 = local read "srateAODOtt"() -> (w1383:dbl)
                    n4573 = local read "continuous"() -> (w1388:bool)
                    n4574 = local read "Angle ref"() -> (w1373:dbl)
                    n4575 = local read "wavdet"() -> (w1390:bool)
                    n4576 = local read "Vx-ref"() -> (w1385:dbl)
                    n4577 = local read "Vy-ref"() -> (w1387:dbl)
                    n4578 = local read "avpp"() -> (w1386:i32)
                    n4579 = call "tt_timeandsamples.vi"("bin"=w1380, "refreshtime"=w1374, "srateAODOtt"=w1377, "tot#ofsamples"=w1382) -> ("refreshrate"=w1378:dbl, "refreshbuffer"=w1379:i32, "timetracecycles"=w1384:i32)  [unwired: 5 in]
                    n4580 = local read "bin"() -> (w1381:dbl)
                    n4581 = call "2pparameters.vi"("command"="get") -> ("params out"=w1393:T11)  [unwired: 1 in]
                    n4582 = Bundle By Name(cluster=w1393, "Drawing Mode"=w1366, "measpoints"=w1382, "tt_cycles"=w1384, "refreshbuffer"=w1379, "refreshrate"=w1378, "Vx-ref"=w1385, "Vy-ref"=w1387, "srate"=w1376, "finite"=w1389, "cont"=w1388, "wavdet"=w1390, "avpp"=w1386, "srateAODO"=w1383, "bufferAI"=w1379, "bin"=w1381, "Angle Img"=w1373, "Vxminref"=w1372, "Vxmaxref"=w1371, "Vyminref"=w1370, "Vymaxref"=w1369, "Xpixels Img"=w1368, "Ypixels Img"=w1367, "Pel"=w1365, "Vz-reset"=0.0, "AIoverride"=w1363, "type"="Lifetime (contour)") -> (w1391:T11)
                    n4583 = Reciprocal(x=w1378) -> (1/x=w1375:dbl)
                    n4584 = local write "refreshtime"(w1375) -> ()
                    n4585 = call "2pparameters.vi"("Params in"=w1391, "command"="set") -> ()  [unwired: 1 out]
                  }
                  frame "X-Y-Z-t movie" {
                  }
                  frame "linescan" {
                  }
                  frame "Timetrace" {
                    n4586 = local read "Vy-min draw"() -> (w1403:dbl)
                    n4587 = local read "Vy-max draw"() -> (w1402:dbl)
                    n4588 = local read "Vx-min draw"() -> (w1405:dbl)
                    n4589 = local read "Vx-max draw"() -> (w1404:dbl)
                    n4590 = local read "xpixels ref"() -> (w1401:i32)
                    n4591 = local read "ypixels ref"() -> (w1400:i32)
                    n4592 = local read "ROI Type"() -> (w1399:u16)
                    n4593 = local read "srateAODOtt"() -> (w1410:dbl)
                    n4594 = local read "# of frames"() -> (w1415:i32)
                    n4595 = local read "refreshtime"() -> (w1407:dbl)
                    n4596 = local read "Pel"() -> (w1398:dbl)
                    n4597 = local read "bin"() -> (w1413:dbl)
                    n4598 = local read "Override AI buffer"() -> (w1396:bool)
                    n4599 = local read "finite samples"() -> (w1422:bool)
                    n4600 = local read "srateAODOtt"() -> (w1409:dbl)
                    n4601 = local read "srateAODOtt"() -> (w1416:dbl)
                    n4602 = local read "continuous"() -> (w1421:bool)
                    n4603 = local read "Angle ref"() -> (w1406:dbl)
                    n4604 = local read "wavdet"() -> (w1423:bool)
                    n4605 = local read "Vx-ref"() -> (w1418:dbl)
                    n4606 = local read "Vy-ref"() -> (w1420:dbl)
                    n4607 = local read "avpp"() -> (w1419:i32)
                    n4608 = call "tt_timeandsamples.vi"("bin"=w1413, "refreshtime"=w1407, "srateAODOtt"=w1410, "tot#ofsamples"=w1415) -> ("refreshrate"=w1411:dbl, "refreshbuffer"=w1412:i32, "timetracecycles"=w1417:i32)  [unwired: 5 in]
                    n4609 = local read "bin"() -> (w1414:dbl)
                    n4610 = call "2pparameters.vi"("command"="get") -> ("params out"=w1426:T11)  [unwired: 1 in]
                    n4611 = Bundle By Name(cluster=w1426, "Drawing Mode"=w1399, "measpoints"=w1415, "tt_cycles"=w1417, "refreshbuffer"=w1412, "refreshrate"=w1411, "Vx-ref"=w1418, "Vy-ref"=w1420, "srate"=w1409, "finite"=w1422, "cont"=w1421, "wavdet"=w1423, "avpp"=w1419, "srateAODO"=w1416, "bufferAI"=w1412, "bin"=w1414, "Angle Img"=w1406, "Vxminref"=w1405, "Vxmaxref"=w1404, "Vyminref"=w1403, "Vymaxref"=w1402, "Xpixels Img"=w1401, "Ypixels Img"=w1400, "Pel"=w1398, "Vz-reset"=0.0, "AIoverride"=w1396, "type"="Timetrace") -> (w1424:T11)
                    n4612 = Reciprocal(x=w1411) -> (1/x=w1408:dbl)
                    n4613 = local write "refreshtime"(w1408) -> ()
                    n4614 = call "2pparameters.vi"("Params in"=w1424, "command"="set") -> ()  [unwired: 1 out]
                  }
                  frame "Lifetime (point)" {
                  }
                }
              }
              frame #1 {
                w1429 = FALSE ("wavdet")
                n4615 = call "2pparameters.vi"("command"="get") -> ("params out"=w1433:T11)  [unwired: 1 in]
                n4616 = Bundle By Name(cluster=w1433, "finite"=w1429, "cont"=w1429, "wavdet"=TRUE) -> (w1430:T11)
                n4617 = call "2pparameters.vi"("Params in"=w1430, "command"="set") -> ()  [unwired: 1 out]
              }
              frame #2 {
                n4618 = local read "AO channels"() -> (w1438:u32)
                n4619 = call "2pparameters.vi"("command"="get") -> ("params out"=w1440:T11)  [unwired: 1 in]
                n4620 = Unbundle By Name(w1440) -> ("aAO"=w1439:u32[])
                n4621 = Search 1D Array(1D array=w1439, element=w1438) -> (index of element=w1436:i32)  [unwired: 1 in]
                n4622 = Greater?(x=w1436, y=-1) -> (0:w1435:bool)
                n4623 = case shown="True" w1435 {
                  tunnel: w1436 -> [_ w1450]
                  frame False {
                  }
                  frame True {
                    n4624 = local read "Meastab"() -> (w1443:enum32{"X-Y Image", "Linescan", "Timetrace"})
                    n4625 = local read "Tri padding value"() -> (w1444:dbl)
                    n4626 = local read "Amplitude (V)"() -> (w1448:dbl)
                    n4627 = local read "Tri Phase (s)"() -> (w1445:dbl)
                    n4628 = local read "Tri Repeats"() -> (w1446:dbl)
                    n4629 = local read "Frequency"() -> (w1447:dbl)
                    n4630 = local read "Offset (V)"() -> (w1449:dbl)
                    n4631 = case shown="\"Timetrace\"" w1443 {
                      tunnel: [w1451 w1452] -> w1442
                      frame "X-Y Image", Default {
                        n4632 = local read "Sampling rate"() -> (w1451:dbl)
                      }
                      frame "Timetrace" {
                        n4633 = local read "srateAODOtt"() -> (w1452:dbl)
                      }
                    }
                    n4634 = call "replace AO tri wf param.vi"("padding value"=w1444, "index of AO wave"=w1450, "Tri phase"=w1445, "Sampling frequency (Hz)"=w1442, "Tri Repeats"=w1446, "Frequency"=w1447, "Amplitude (V)"=w1448, "Offset (V)"=w1449) -> ()
                  }
                }
              }
              frame #3 {
                n4635 = case shown="True" w1453 {
                  tunnel: w1454 -> [_ w1463]
                  frame False {
                  }
                  frame True {
                    n4636 = call "waveformparamsv2.vi"("command"="get") -> ("Params out"=w1476:T15)  [unwired: 4 in, 2 out]
                    n4637 = Unbundle By Name(w1476) -> ("AO parameters"=w1475:T16)
                    n4638 = local read "Meastab"() -> (w1458:enum32{"X-Y Image", "Linescan", "Timetrace"})
                    n4639 = case shown="\"Timetrace\"" w1458 {
                      tunnel: [w1478 w1479] -> w1457
                      frame "X-Y Image", Default {
                        n4640 = local read "Sampling rate"() -> (w1478:dbl)
                      }
                      frame "Timetrace" {
                        n4641 = local read "srateAODOtt"() -> (w1479:dbl)
                      }
                    }
                    n4642 = Index Array(array=w1475, index=w1463) -> (element=w1465:T17)
                    n4643 = call "waveformsAObuffer.vi"("command"="get") -> ("AO wf out"=w1464:waveform(dbl)[])  [unwired: 1 in]
                    n4644 = call "generateTriWave_fromAOparameters.vi"("AO params"=w1465) -> ("Waveform"=w1462:waveform(dbl))  [unwired: 1 out]
                    n4645 = property on="refwf" class="Ring (strict)"() -> ("RingText.Text"=w1466:string)  [unwired: 2 in, 2 out]
                    n4646 = Replace Array Subset(array=w1464, new element=w1462, index=w1463) -> (w1461:waveform(dbl)[])
                    n4647 = call "waveformsDObuffer.vi"("command"="get") -> ("DO wf out"=w1471:digitalwaveform[])  [unwired: 1 in]
                    n4648 = call "correctwaveformsizetemp.vi"("new sampling frequency (Hz)"=w1457, "start"=FALSE, "reference waveforms to"=w1466, "Analog waveforms in"=w1461, "stop"=FALSE, "Digital waveforms in"=w1471) -> ("analog wf out"=w1469:waveform(dbl)[], "Digital wf out"=w1467:digitalwaveform[], "measpoints"=w1459:i32)
                    n4649 = local read "wavdet"() -> (w1460:bool)
                    n4650 = local write "Analog Lines Plot"(w1469) -> ()
                    n4651 = call "GetNumCamFramesv2.vi"("Digital Waveform Graph"=w1467) -> ("Numeric"=w1468:i32)  [unwired: 10 in]
                    n4652 = local write "Digital Lines Plot"(w1467) -> ()
                    n4653 = call "waveformsAObuffer.vi"("AO wf in"=w1469, "command"="set") -> ()  [unwired: 1 out]
                    n4654 = call "waveformsDObuffer.vi"("DO wf in"=w1467, "command"="set") -> ()  [unwired: 1 out]
                    n4655 = local write "Total Camera Frames"(w1468) -> ()
                    n4656 = case shown="True" w1460 {
                      tunnel: w1459 -> [_ w1480]
                      frame False {
                      }
                      frame True {
                        n4657 = local write "# of frames"(w1480) -> ()
                      }
                    }
                  }
                }
              }
              frame #4 {
                n4658 = local read "finite samples"() -> (w1481:bool)
                n4659 = local read "continuous"() -> (w1482:bool)
                n4660 = local read "wavdet"() -> (w1483:bool)
                n4661 = call "2pparameters.vi"("command"="get") -> ("params out"=w1486:T11)  [unwired: 1 in]
                n4662 = Bundle By Name(cluster=w1486, "finite"=w1481, "cont"=w1482, "wavdet"=w1483) -> (w1484:T11)
                n4663 = call "2pparameters.vi"("Params in"=w1484, "command"="set") -> ()  [unwired: 1 out]
              }
            }
          }
          event "Load Matlab Waveform": Value Change {
            n4664 = event-data() -> ()  [unwired: 1 in, 6 out]
            n4665 = stacked-sequence {
              seq-local: [_ _ w1594 _ _] -> [_ _ _ w1609 _]
              seq-local: [_ _ w1593 _ _] -> [_ _ _ w1608 _]
              frame #0 {
                n4666 = local read "Measurement"() -> (w1488:T4)
                n4667 = case shown="\"X-Y-t movie\", Default" w1488 {
                  frame "X-Y-t movie", Default {
                    n4668 = local read "avpp"() -> (w1509:i32)
                    n4669 = local read "Angle ref"() -> (w1508:dbl)
                    n4670 = local read "ROI Type"() -> (w1507:u16)
                    n4671 = local read "xpixels ref"() -> (w1504:i32)
                    n4672 = local read "Vx-min ref"() -> (w1503:dbl)
                    n4673 = local read "Vx-max ref"() -> (w1502:dbl)
                    n4674 = local read "ypixels ref"() -> (w1500:i32)
                    n4675 = local read "Vy-min ref"() -> (w1501:dbl)
                    n4676 = local read "Vy-max ref"() -> (w1497:dbl)
                    n4677 = local read "Sampling rate"() -> (w1491:dbl)
                    n4678 = local read "finite samples"() -> (w1492:bool)
                    n4679 = local read "continuous"() -> (w1495:bool)
                    n4680 = local read "wavdet"() -> (w1496:bool)
                    n4681 = local read "# of frames"() -> (w1494:i32)
                    n4682 = local read "maxbufferAI"() -> (w1493:i32)
                    n4683 = local read "Override AI buffer"() -> (w1489:bool)
                    n4684 = call "2pparameters.vi"("command"="get") -> ("params out"=w1506:T11)  [unwired: 1 in]
                    n4685 = Bundle By Name(cluster=w1506, "type"="X-Y-t movie", "avpp"=w1509, "Angle Img"=w1508, "Xpixels Img"=w1504, "Vx-min Img"=w1503, "VX-max Img"=w1502, "Ypixels Img"=w1500, "Vy-min Img"=w1501, "Vy-max Img"=w1497, "srate"=w1491, "srate Img"=w1491, "finite"=w1492, "cont"=w1495, "wavdet"=w1496, "measpoints"=w1494, "maxbufferAI"=w1493, "Drawing Mode"=w1507, "Vz-reset"=0.0, "AIoverride"=w1489) -> (w1498:T11)
                    n4686 = call "2pparameters.vi"("Params in"=w1498, "command"="set") -> ()  [unwired: 1 out]
                  }
                  frame "X-Y-Z stack" {
                    n4687 = call "2pparameters.vi"("command"="get") -> ("params out"=w1513:T11)  [unwired: 1 in]
                    n4688 = Bundle By Name(cluster=w1513, "type"="X-Y-Z stack") -> (w1511:T11)
                    n4689 = call "2pparameters.vi"("Params in"=w1511, "command"="set") -> ()  [unwired: 1 out]
                  }
                  frame "Lifetime (scan)" {
                    n4690 = call "2pparameters.vi"("command"="get") -> ("params out"=w1518:T11)  [unwired: 1 in]
                    n4691 = Bundle By Name(cluster=w1518, "type"="Lifetime (scan)") -> (w1516:T11)
                    n4692 = call "2pparameters.vi"("Params in"=w1516, "command"="set") -> ()  [unwired: 1 out]
                  }
                  frame "Lifetime (contour)" {
                    n4693 = local read "Vy-min draw"() -> (w1528:dbl)
                    n4694 = local read "Vy-max draw"() -> (w1527:dbl)
                    n4695 = local read "Vx-min draw"() -> (w1530:dbl)
                    n4696 = local read "Vx-max draw"() -> (w1529:dbl)
                    n4697 = local read "xpixels ref"() -> (w1526:i32)
                    n4698 = local read "ypixels ref"() -> (w1525:i32)
                    n4699 = local read "ROI Type"() -> (w1524:u16)
                    n4700 = local read "srateAODOtt"() -> (w1535:dbl)
                    n4701 = local read "# of frames"() -> (w1540:i32)
                    n4702 = local read "refreshtime"() -> (w1532:dbl)
                    n4703 = local read "Pel"() -> (w1523:dbl)
                    n4704 = local read "bin"() -> (w1538:dbl)
                    n4705 = local read "Override AI buffer"() -> (w1521:bool)
                    n4706 = local read "finite samples"() -> (w1547:bool)
                    n4707 = local read "srateAODOtt"() -> (w1534:dbl)
                    n4708 = local read "srateAODOtt"() -> (w1541:dbl)
                    n4709 = local read "continuous"() -> (w1546:bool)
                    n4710 = local read "Angle ref"() -> (w1531:dbl)
                    n4711 = local read "wavdet"() -> (w1548:bool)
                    n4712 = local read "Vx-ref"() -> (w1543:dbl)
                    n4713 = local read "Vy-ref"() -> (w1545:dbl)
                    n4714 = local read "avpp"() -> (w1544:i32)
                    n4715 = call "tt_timeandsamples.vi"("bin"=w1538, "refreshtime"=w1532, "srateAODOtt"=w1535, "tot#ofsamples"=w1540) -> ("refreshrate"=w1536:dbl, "refreshbuffer"=w1537:i32, "timetracecycles"=w1542:i32)  [unwired: 5 in]
                    n4716 = local read "bin"() -> (w1539:dbl)
                    n4717 = call "2pparameters.vi"("command"="get") -> ("params out"=w1551:T11)  [unwired: 1 in]
                    n4718 = Bundle By Name(cluster=w1551, "Drawing Mode"=w1524, "measpoints"=w1540, "tt_cycles"=w1542, "refreshbuffer"=w1537, "refreshrate"=w1536, "Vx-ref"=w1543, "Vy-ref"=w1545, "srate"=w1534, "finite"=w1547, "cont"=w1546, "wavdet"=w1548, "avpp"=w1544, "srateAODO"=w1541, "bufferAI"=w1537, "bin"=w1539, "Angle Img"=w1531, "Vxminref"=w1530, "Vxmaxref"=w1529, "Vyminref"=w1528, "Vymaxref"=w1527, "Xpixels Img"=w1526, "Ypixels Img"=w1525, "Pel"=w1523, "Vz-reset"=0.0, "AIoverride"=w1521, "type"="Lifetime (contour)") -> (w1549:T11)
                    n4719 = Reciprocal(x=w1536) -> (1/x=w1533:dbl)
                    n4720 = local write "refreshtime"(w1533) -> ()
                    n4721 = call "2pparameters.vi"("Params in"=w1549, "command"="set") -> ()  [unwired: 1 out]
                  }
                  frame "X-Y-Z-t movie" {
                  }
                  frame "linescan" {
                  }
                  frame "Timetrace" {
                    n4722 = local read "Vy-min draw"() -> (w1561:dbl)
                    n4723 = local read "Vy-max draw"() -> (w1560:dbl)
                    n4724 = local read "Vx-min draw"() -> (w1563:dbl)
                    n4725 = local read "Vx-max draw"() -> (w1562:dbl)
                    n4726 = local read "xpixels ref"() -> (w1559:i32)
                    n4727 = local read "ypixels ref"() -> (w1558:i32)
                    n4728 = local read "ROI Type"() -> (w1557:u16)
                    n4729 = local read "srateAODOtt"() -> (w1568:dbl)
                    n4730 = local read "# of frames"() -> (w1573:i32)
                    n4731 = local read "refreshtime"() -> (w1565:dbl)
                    n4732 = local read "Pel"() -> (w1556:dbl)
                    n4733 = local read "bin"() -> (w1571:dbl)
                    n4734 = local read "Override AI buffer"() -> (w1554:bool)
                    n4735 = local read "finite samples"() -> (w1580:bool)
                    n4736 = local read "srateAODOtt"() -> (w1567:dbl)
                    n4737 = local read "srateAODOtt"() -> (w1574:dbl)
                    n4738 = local read "continuous"() -> (w1579:bool)
                    n4739 = local read "Angle ref"() -> (w1564:dbl)
                    n4740 = local read "wavdet"() -> (w1581:bool)
                    n4741 = local read "Vx-ref"() -> (w1576:dbl)
                    n4742 = local read "Vy-ref"() -> (w1578:dbl)
                    n4743 = local read "avpp"() -> (w1577:i32)
                    n4744 = call "tt_timeandsamples.vi"("bin"=w1571, "refreshtime"=w1565, "srateAODOtt"=w1568, "tot#ofsamples"=w1573) -> ("refreshrate"=w1569:dbl, "refreshbuffer"=w1570:i32, "timetracecycles"=w1575:i32)  [unwired: 5 in]
                    n4745 = local read "bin"() -> (w1572:dbl)
                    n4746 = call "2pparameters.vi"("command"="get") -> ("params out"=w1584:T11)  [unwired: 1 in]
                    n4747 = Bundle By Name(cluster=w1584, "Drawing Mode"=w1557, "measpoints"=w1573, "tt_cycles"=w1575, "refreshbuffer"=w1570, "refreshrate"=w1569, "Vx-ref"=w1576, "Vy-ref"=w1578, "srate"=w1567, "finite"=w1580, "cont"=w1579, "wavdet"=w1581, "avpp"=w1577, "srateAODO"=w1574, "bufferAI"=w1570, "bin"=w1572, "Angle Img"=w1564, "Vxminref"=w1563, "Vxmaxref"=w1562, "Vyminref"=w1561, "Vymaxref"=w1560, "Xpixels Img"=w1559, "Ypixels Img"=w1558, "Pel"=w1556, "Vz-reset"=0.0, "AIoverride"=w1554, "type"="Timetrace") -> (w1582:T11)
                    n4748 = Reciprocal(x=w1569) -> (1/x=w1566:dbl)
                    n4749 = local write "refreshtime"(w1566) -> ()
                    n4750 = call "2pparameters.vi"("Params in"=w1582, "command"="set") -> ()  [unwired: 1 out]
                  }
                  frame "Lifetime (point)" {
                  }
                }
              }
              frame #1 {
                w1587 = FALSE ("wavdet")
                n4751 = call "2pparameters.vi"("command"="get") -> ("params out"=w1591:T11)  [unwired: 1 in]
                n4752 = Bundle By Name(cluster=w1591, "finite"=w1587, "cont"=w1587, "wavdet"=TRUE) -> (w1588:T11)
                n4753 = call "2pparameters.vi"("Params in"=w1588, "command"="set") -> ()  [unwired: 1 out]
              }
              frame #2 {
                n4754 = local read "AO channels"() -> (w1596:u32)
                n4755 = call "2pparameters.vi"("command"="get") -> ("params out"=w1598:T11)  [unwired: 1 in]
                n4756 = Unbundle By Name(w1598) -> ("aAO"=w1597:u32[])
                n4757 = Search 1D Array(1D array=w1597, element=w1596) -> (index of element=w1594:i32)  [unwired: 1 in]
                n4758 = Greater?(x=w1594, y=-1) -> (0:w1593:bool)
                n4759 = case shown="True" w1593 {
                  tunnel: w1594 -> [_ w1605]
                  frame False {
                  }
                  frame True {
                    n4760 = local read "Meastab"() -> (w1601:enum32{"X-Y Image", "Linescan", "Timetrace"})
                    n4761 = local read "Matlab waveform path"() -> (w1603:path)
                    n4762 = local read "Matlab padding value"() -> (w1604:dbl)
                    n4763 = case shown="\"Timetrace\"" w1601 {
                      tunnel: [w1606 w1607] -> w1600
                      frame "X-Y Image", Default {
                        n4764 = local read "Sampling rate"() -> (w1606:dbl)
                      }
                      frame "Timetrace" {
                        n4765 = local read "srateAODOtt"() -> (w1607:dbl)
                      }
                    }
                    n4766 = call "matlabwfexistsdialogue.vi"("Matlab waveform path"=w1603) -> ("mtalab waveform path out"=w1602:path)
                    n4767 = call "replace AO matlab param.vi"("Sampling frequency (Hz)"=w1600, "matlab wave file"=w1602, "index of AO wave"=w1605, "padding value"=w1604) -> ()  [unwired: 7 in]
                  }
                }
              }
              frame #3 {
                n4768 = case shown="True" w1608 {
                  tunnel: w1609 -> [_ w1616]
